vi "New.vi"() -> ()   [LabVIEW 2019]
uses:
  C:/Program Files (x86)/National Instruments/LabVIEW 2019/examples/Design Patterns/Queued Message Handler/support/QMH Fundamentals - Message Cluster.ctl
  81650588-77ff-4ea7-96b2-54a9c01bfe74.vi
panel:
  out "Artificial Data Dependence":bool
  in  "Make Visible?":bool
  in  "Developer Settings":bool
  in  "Match Ready":bool
  in  "Left Sidebar Expanded":bool
  in  "Flywheel Velocity":i32
  out "Numeric 2":dbl
  out "Highest Temp Label":string
  in  "Right Lead":dbl(slide) scale=0.0..100.0
  in  "Left Follow":dbl(slide) scale=0.0..100.0
  in  "Left Lead":dbl(slide) scale=0.0..100.0
  in  "stop 2":bool
  in  "Left Sidebar Mini":bool
  in  "stop":bool
  out "Widger Manager":enum32{"Page 1", "Page 2"}(tab)
  out "String 3":string
  out "String 2":string
  in  "Boolean 3":bool
  in  "Boolean 2":bool
  out "# elements in queue 2":i32
  out "Elapsed Time (s)":dbl
  out "# elements in queue":i32
  in  "Turret Value":string
  in  "Exanded View Toolbar":bool
  in  "Mini View Button":bool
  in  "Mini View Toolbar":bool
  in  "Shooter Value":string
  in  "Minimized Toolbar Button":bool
  out "String":string
  out "Boolean 5":bool
  in  "Robot Connection":bool
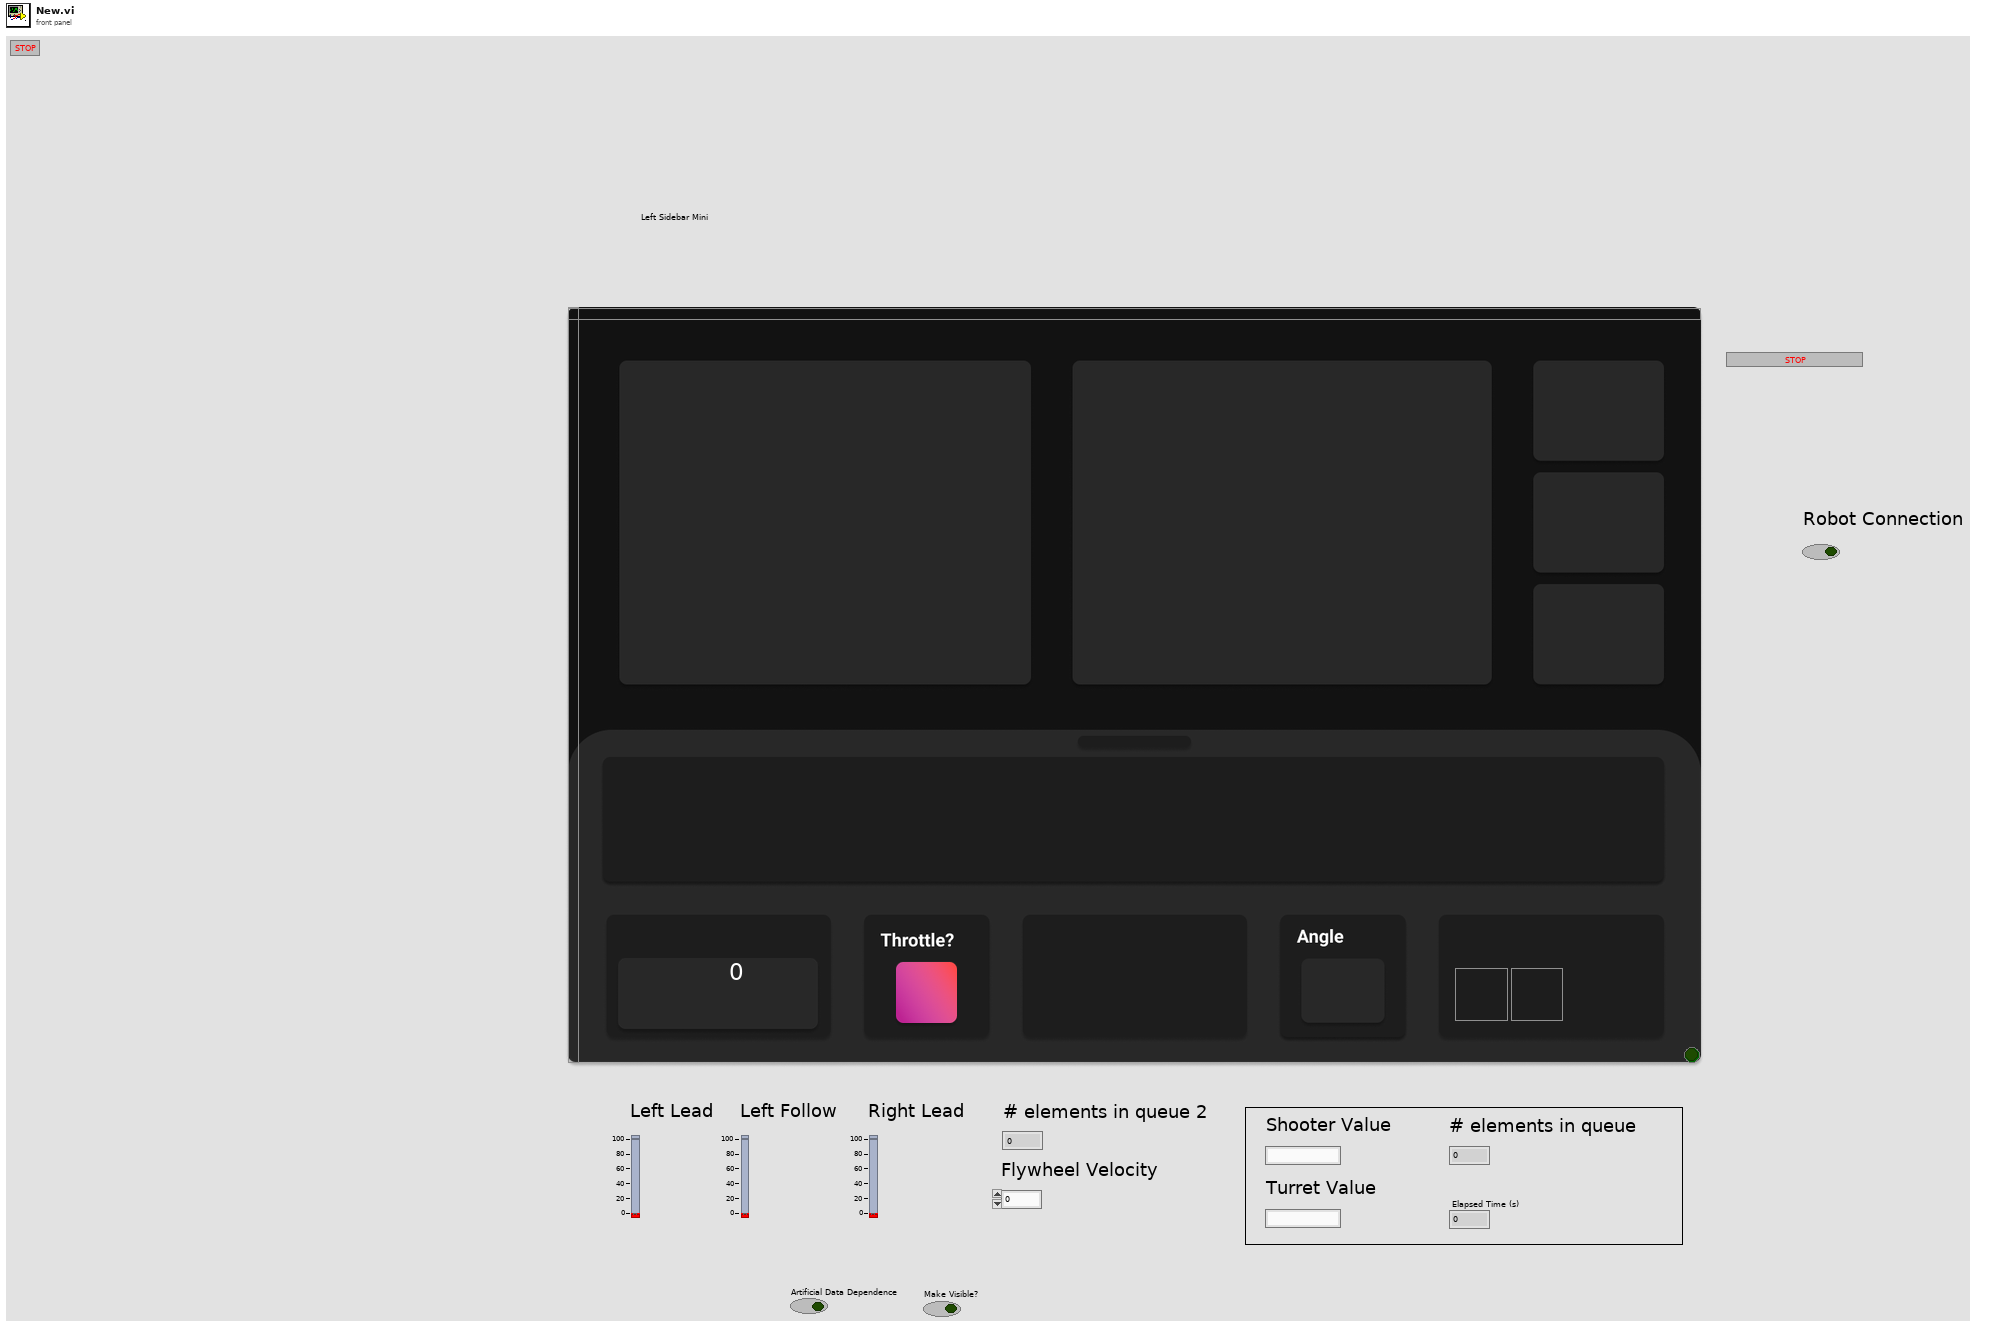
[diagram p1: front panel]
types:
  T1 = typedef "QMH Fundamentals - Message Cluster.ctl" = cluster{"Message":string, "Message Data":variant, "Time":timestamp}
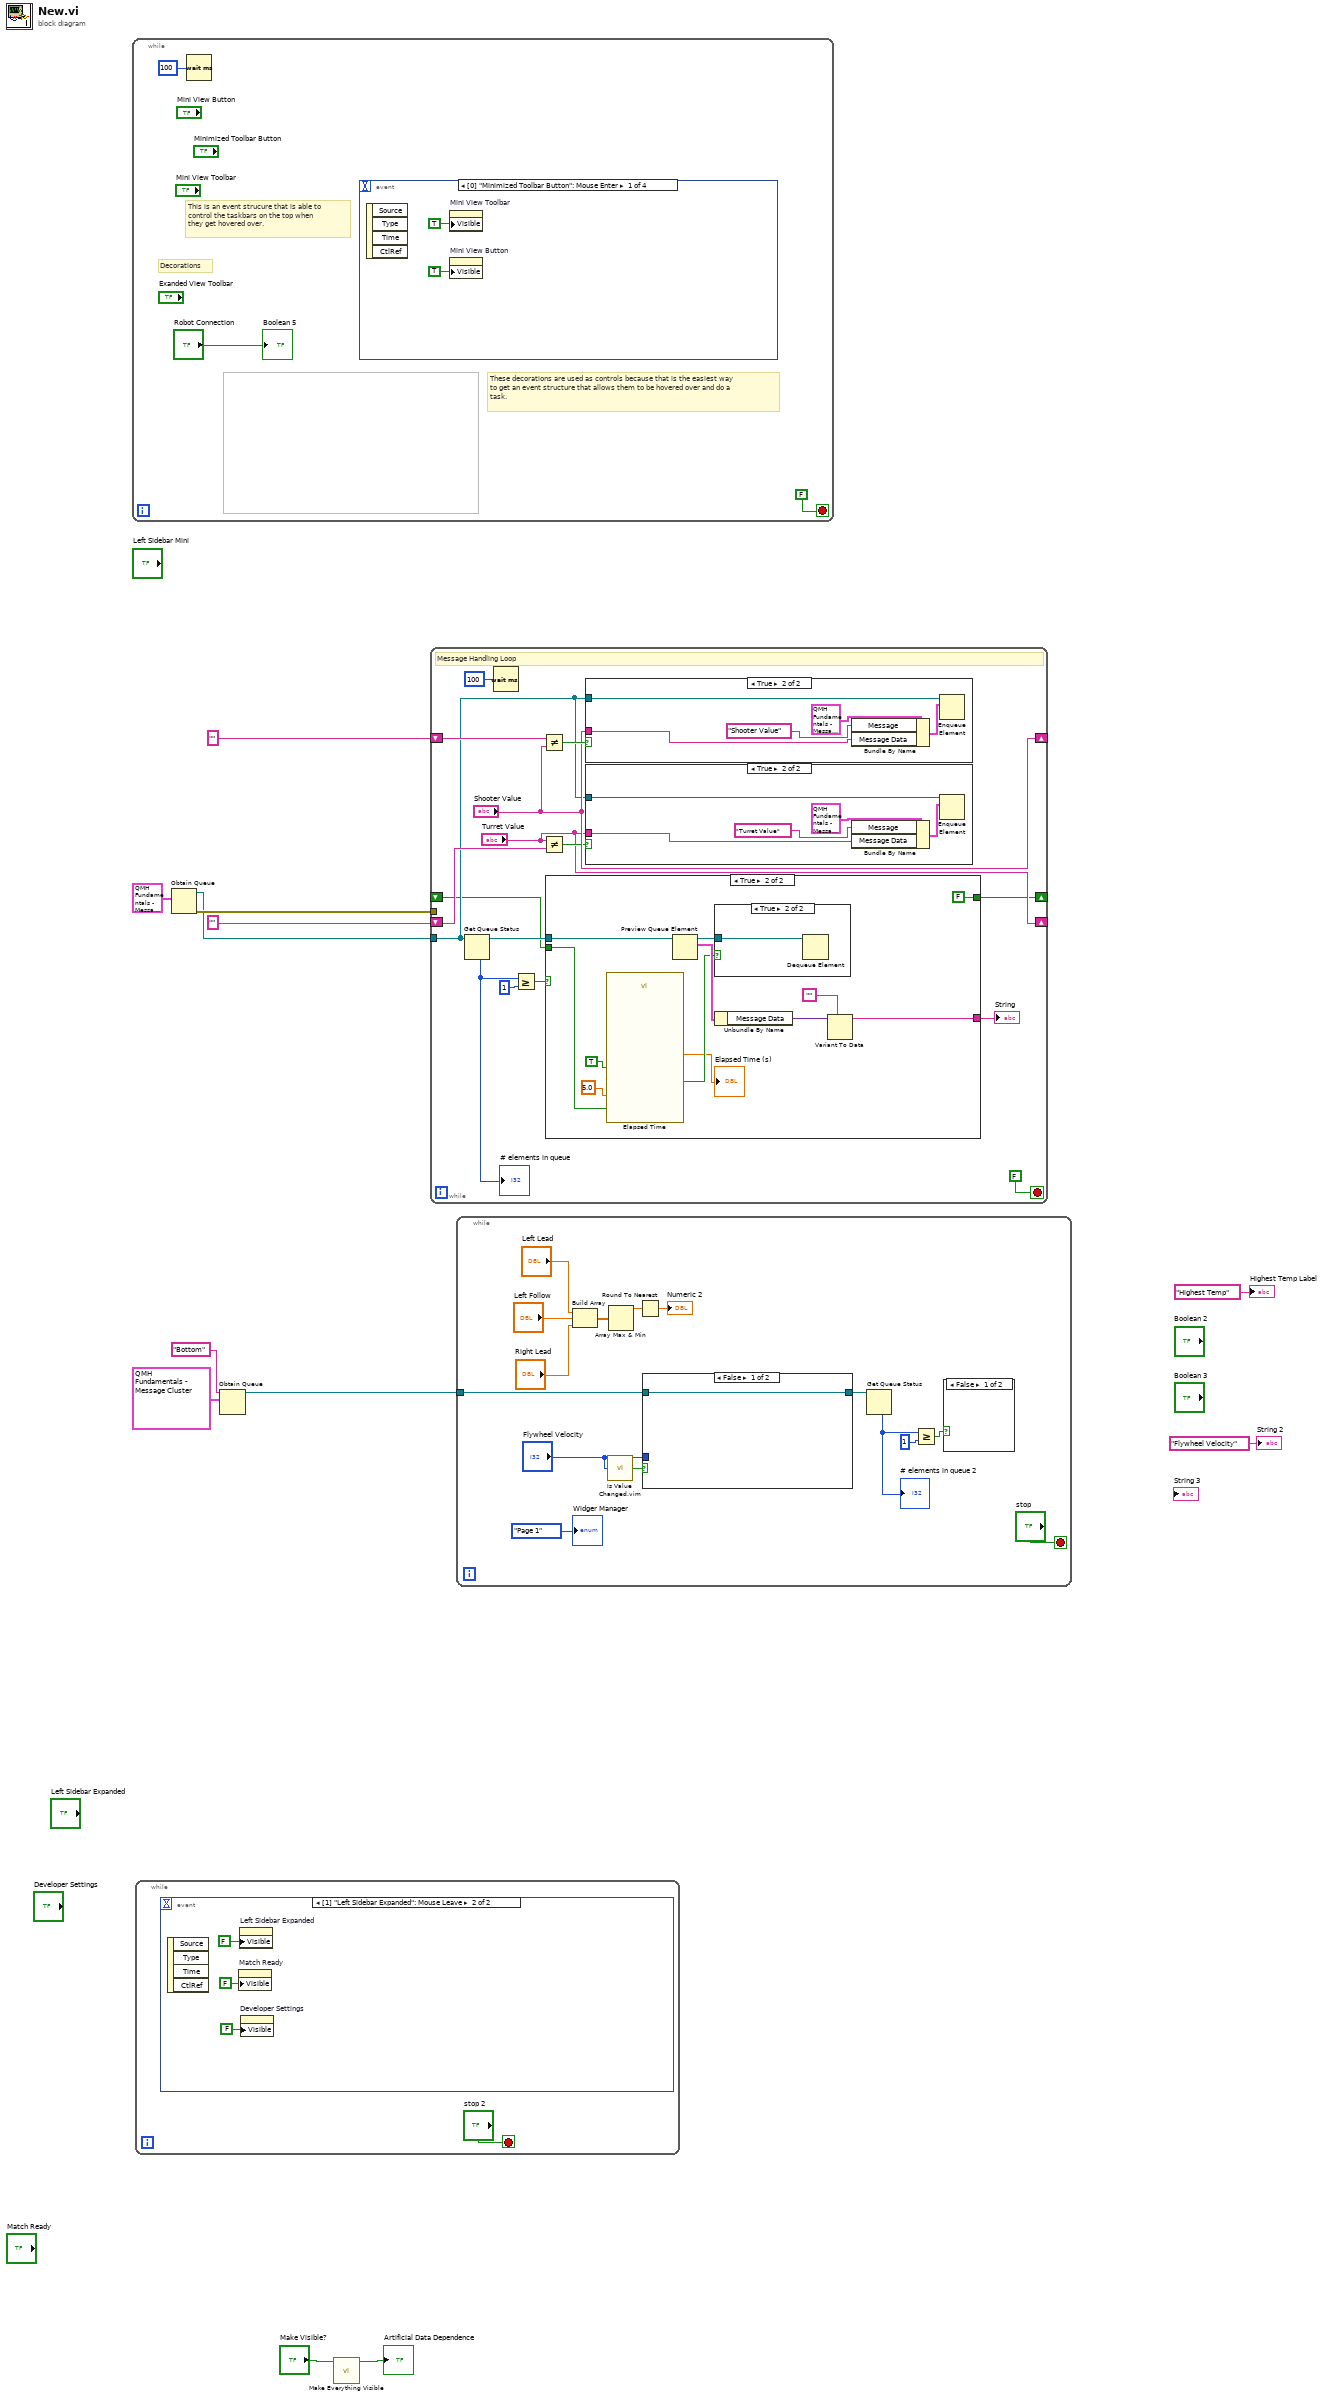
[diagram p0: block diagram]
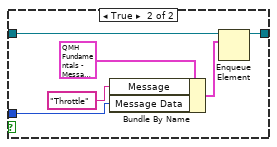
[diagram p2: hidden frame]
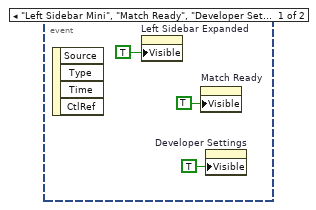
[diagram p4: hidden frame]
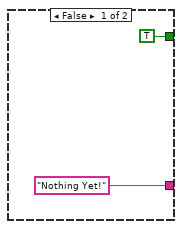
[diagram p5: hidden frame]
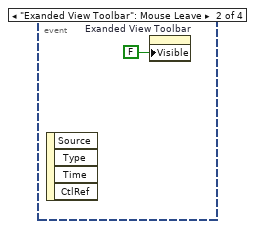
[diagram p9: hidden frame]
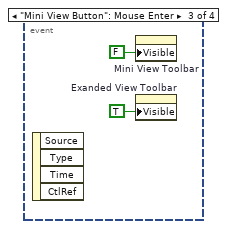
[diagram p10: hidden frame]
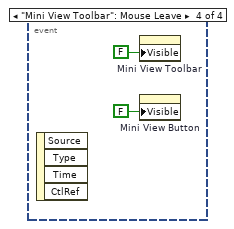
[diagram p11: hidden frame]
diagram:
  n1 = while {
    stop <- FALSE stop-if-true
    # "This is an event strucure that is able to\ncontrol the taskbars on the top when \nthey get hovered over."
    # "These decorations are used as controls because that is the easiest way to get an event structure that allows them to be hovered over and do a task."
    # "Decorations"
    n2 = Wait (ms)(milliseconds to wait=u32 100) -> ()  [unwired: 1 out]
    n3 = event shown="[0] \"Minimized Toolbar Button\": Mouse Enter" {
      selector: _ -> [_ _ _ _]
      dyn-events: _ -> [_ _ _ _]
      timeout: _ -> [_ _ _ _]
      event "Minimized Toolbar Button": Mouse Enter {
        n4 = event-data() -> ()  [unwired: 1 in, 4 out]
        n5 = property on="Mini View Toolbar" class="Bool (strict)"("Visible"=TRUE) -> ()  [unwired: 2 in, 2 out]
        n6 = property on="Mini View Button" class="Bool (strict)"("Visible"=TRUE) -> ()  [unwired: 2 in, 2 out]
      }
      event "Exanded View Toolbar": Mouse Leave {
        n7 = event-data() -> ()  [unwired: 1 in, 4 out]
        n8 = property on="Exanded View Toolbar" class="Bool (strict)"("Visible"=FALSE) -> ()  [unwired: 2 in, 2 out]
      }
      event "Mini View Button": Mouse Enter {
        n9 = event-data() -> ()  [unwired: 1 in, 4 out]
        n10 = property on="Mini View Toolbar" class="Bool (strict)"("Visible"=FALSE) -> ()  [unwired: 2 in, 2 out]
        n11 = property on="Exanded View Toolbar" class="Bool (strict)"("Visible"=TRUE) -> ()  [unwired: 2 in, 2 out]
      }
      event "Mini View Toolbar": Mouse Leave {
        n12 = event-data() -> ()  [unwired: 1 in, 4 out]
        n13 = property on="Mini View Toolbar" class="Bool (strict)"("Visible"=FALSE) -> ()  [unwired: 2 in, 2 out]
        n14 = property on="Mini View Button" class="Bool (strict)"("Visible"=FALSE) -> ()  [unwired: 2 in, 2 out]
      }
    }
    "Boolean 5" <- "Robot Connection"
  }
  n15 = while {
    stop <- "stop 2" stop-if-true
    n16 = event shown="[1] \"Left Sidebar Expanded\": Mouse Leave" {
      selector: _ -> [_ _]
      dyn-events: _ -> [_ _]
      timeout: _ -> [_ _]
      event "Left Sidebar Mini", "Match Ready", "Developer Settings": Mouse Enter {
        n17 = event-data() -> ()  [unwired: 1 in, 4 out]
        n18 = property on="Left Sidebar Expanded" class="Bool (strict)"("Visible"=TRUE) -> ()  [unwired: 2 in, 2 out]
        n19 = property on="Match Ready" class="Bool (strict)"("Visible"=TRUE) -> ()  [unwired: 2 in, 2 out]
        n20 = property on="Developer Settings" class="Bool (strict)"("Visible"=TRUE) -> ()  [unwired: 2 in, 2 out]
      }
      event "Left Sidebar Expanded": Mouse Leave {
        n21 = event-data() -> ()  [unwired: 1 in, 4 out]
        n22 = property on="Match Ready" class="Bool (strict)"("Visible"=FALSE) -> ()  [unwired: 2 in, 2 out]
        n23 = property on="Left Sidebar Expanded" class="Bool (strict)"("Visible"=FALSE) -> ()  [unwired: 2 in, 2 out]
        n24 = property on="Developer Settings" class="Bool (strict)"("Visible"=FALSE) -> ()  [unwired: 2 in, 2 out]
      }
    }
  }
  n25 = Obtain Queue(element data type=T1 {"Message"="", "Message Data"=variant, "Time"=timestamp(0 s since 1904-01-01)} ("Message Cluster")) -> (queue out=w8:refnum<queue>, error out=w9:errorcluster)  [unwired: 4 in, 1 out]
  n26 = Obtain Queue(name (unnamed)="Bottom", element data type=T1 {"Message"="", "Message Data"=variant, "Time"=timestamp(0 s since 1904-01-01)} ("Message Cluster")) -> (queue out=w3:refnum<queue>)  [unwired: 3 in, 2 out]
  n27 = call "Make Everything Visible.vi"("Make Visible?"="Make Visible?") -> ("Artificial Data Dependence"=→"Artificial Data Dependence":bool)  [unwired: 10 in]
  n28 = while {
    tunnel: w9 -> [_]
    tunnel: w8 -> [w39]
    shift-right: ["Shooter Value"] -> _
    shift-left: "" -> [w44]
    shift-right: ["Turret Value"] -> _
    shift-left: "" -> [w41]
    shift-right: [w32] -> _
    shift-left: _ -> [w31]
    stop <- FALSE stop-if-true
    # "Message Handling Loop"
    n29 = Get Queue Status(queue=w39) -> (queue out=w34:refnum<queue>, # elements in queue=w37:i32)  [unwired: 2 in, 6 out]
    "# elements in queue" <- w37
    n30 = Wait (ms)(milliseconds to wait=u32 100) -> ()  [unwired: 1 out]
    n31 = Greater Or Equal?(x=w37, y=1) -> (x >= y?=w35:bool)
    n32 = Not Equal?(x=w44, y="Shooter Value") -> (x != y?=w43:bool)
    n33 = Not Equal?(x="Turret Value", y=w41) -> (x != y?=w40:bool)
    n34 = case shown="True" w35 {
      tunnel: ["Nothing Yet!" w58] -> w30
      tunnel: w34 -> [_ w56]
      tunnel: [TRUE FALSE ("Auto Reset")] -> w32
      tunnel: w31 -> [_ w48]
      frame False {
      }
      frame True {
        n35 = call "Elapsed Time"("Time Target (s)"=5.0, "Reset"=w48, "Auto Reset"=TRUE) -> ("Elapsed Time (s)"=→"Elapsed Time (s)":dbl, "Time has Elapsed"=w51:bool)  [unwired: 9 in, 6 out]
        n36 = Preview Queue Element(queue=w56) -> (queue out=w54:refnum<queue>, element=w55:T1)  [unwired: 2 in, 2 out]
        n37 = case shown="True" w51 {
          tunnel: w54 -> [_ w60]
          frame False {
          }
          frame True {
            n38 = Dequeue Element(queue=w60) -> ()  [unwired: 2 in, 4 out]
          }
        }
        n39 = Unbundle By Name(w55) -> ("Message Data"=w57:variant)
        n40 = Variant To Data(type="", Variant=w57) -> (data=w58:string)  [unwired: 1 in, 1 out]
      }
    }
    "String" <- w30
    n41 = case shown="True" w43 {
      tunnel: w39 -> [_ w67]
      tunnel: "Shooter Value" -> [_ w66]
      frame False {
      }
      frame True {
        n42 = Bundle By Name(cluster=T1 {"Message"="", "Message Data"=variant, "Time"=timestamp(0 s since 1904-01-01)} ("element"), "Message"="Shooter Value", "Message Data"=w66) -> (w70:T1)
        n43 = Enqueue Element(queue=w67, element=w70) -> ()  [unwired: 2 in, 3 out]
      }
    }
    n44 = case shown="True" w40 {
      tunnel: "Turret Value" -> [_ w62]
      tunnel: w39 -> [_ w61]
      frame False {
      }
      frame True {
        n45 = Bundle By Name(cluster=T1 {"Message"="", "Message Data"=variant, "Time"=timestamp(0 s since 1904-01-01)} ("element"), "Message"="Turret Value", "Message Data"=w62) -> (w65:T1)
        n46 = Enqueue Element(queue=w61, element=w65) -> ()  [unwired: 2 in, 3 out]
      }
    }
  }
  n47 = while {
    tunnel: w3 -> [w75]
    stop <- "stop" stop-if-true
    n48 = Build Array("Left Lead", "Left Follow", "Right Lead") -> (w78:dbl[])
    n49 = call "Is Value Changed.vim"("value"="Flywheel Velocity") -> ("changed or first call?"=w77:bool)
    n50 = Array Max & Min(array=w78) -> (max value=w72:dbl)  [unwired: 3 out]
    n51 = Round To Nearest(number=w72) -> (nearest integer value=→"Numeric 2":dbl)
    n52 = case shown="False" w77 {
      tunnel: "Flywheel Velocity" -> [_ w89]
      tunnel: w75 -> [w86 w88]
      tunnel: [w86 w87] -> w74
      frame False {
      }
      frame True {
        n53 = Bundle By Name(cluster=T1 {"Message"="", "Message Data"=variant, "Time"=timestamp(0 s since 1904-01-01)} ("element"), "Message"="Throttle", "Message Data"=w89) -> (w92:T1)
        n54 = Enqueue Element(queue=w88, element=w92) -> (queue out=w87:refnum<queue>)  [unwired: 2 in, 2 out]
      }
    }
    n55 = Get Queue Status(queue=w74) -> (# elements in queue=w82:i32)  [unwired: 2 in, 7 out]
    "# elements in queue 2" <- w82
    n56 = Greater Or Equal?(x=w82, y=1) -> (x >= y?=w84:bool)
    n57 = case shown="False" w84 {
      frame False {
      }
      frame True {
      }
    }
    "Widger Manager" <- enum32{"Page 1", "Page 2"}."Page 1" ("Widger Manager")
  }
  "Highest Temp Label" <- "Highest Temp" ("Highest Temp Label")
  "String 2" <- "Flywheel Velocity" ("String 2")
